vi "Trigger 2.vi"() -> ()   [LabVIEW 2012]
panel:
  in  "CO2 ppm":dbl(slide)
  in  "CO2 Trigger":T1={"Boost A Threshold"=0.0, "Boost A Hyst"=-250.0, "Boost B Threshold"=50.0, "Boost B Hyst"=-150.0}
  out "Alt Diff Down":bool
  out "Alt Dif Last":dbl
  out "Alt States":T2={"Main"=TRUE, "Boost A"=FALSE, "Boost B"=FALSE, "Recirc"=FALSE, "Scrubber"=FALSE, "O2 Valve"=FALSE, "Vent"=FALSE, "Alarm"=FALSE}
  in  "Alt Dif":dbl(slide) scale=-1000.0..1000.0
  in  "Stop Progam":bool
  out "Loops":i32
  in  "Alt Trigger":T3={"Boost A Threshold"=0.0, "Boost A Hyst"=-250.0, "Boost B Threshold"=50.0, "Boost B Hyst"=-150.0, "O2 Threshold"=250.0, "O2 Hyst"=400.0, "Vent Threshold"=50.0, "Vent Hyst"=200.0, "Recirc Threshold "=50.0, "Recirc  Hyst "=-150.0}
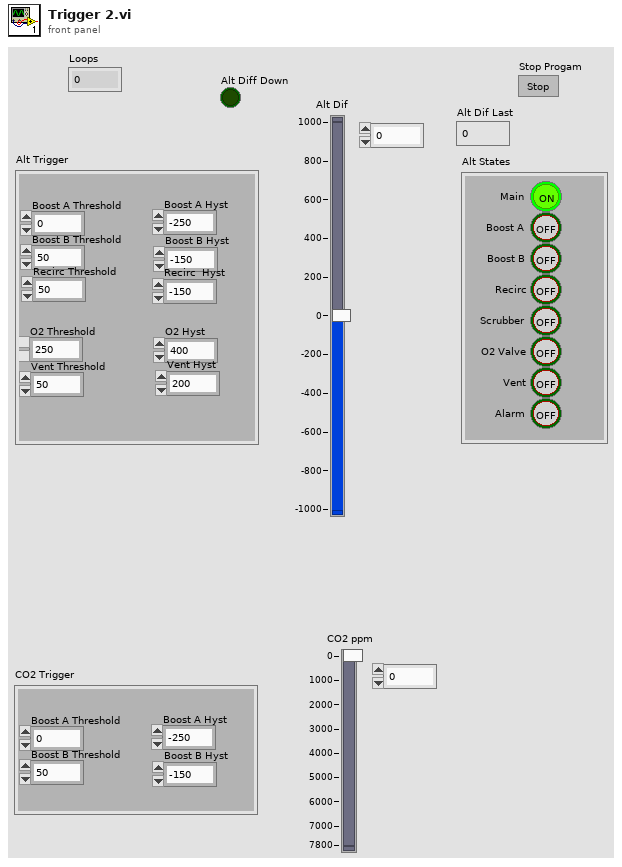
[diagram p1: front panel]
types:
  T1 = cluster{"Boost A Threshold":dbl, "Boost A Hyst":dbl, "Boost B Threshold":dbl, "Boost B Hyst":dbl}
  T2 = cluster{"Main":bool, "Boost A":bool, "Boost B":bool, "Recirc":bool, "Scrubber":bool, "O2 Valve":bool, "Vent":bool, "Alarm":bool}
  T3 = cluster{"Boost A Threshold":dbl, "Boost A Hyst":dbl, "Boost B Threshold":dbl, "Boost B Hyst":dbl, "O2 Threshold":dbl, "O2 Hyst":dbl, "Vent Threshold":dbl, "Vent Hyst":dbl, "Recirc Threshold ":dbl, "Recirc  Hyst ":dbl}
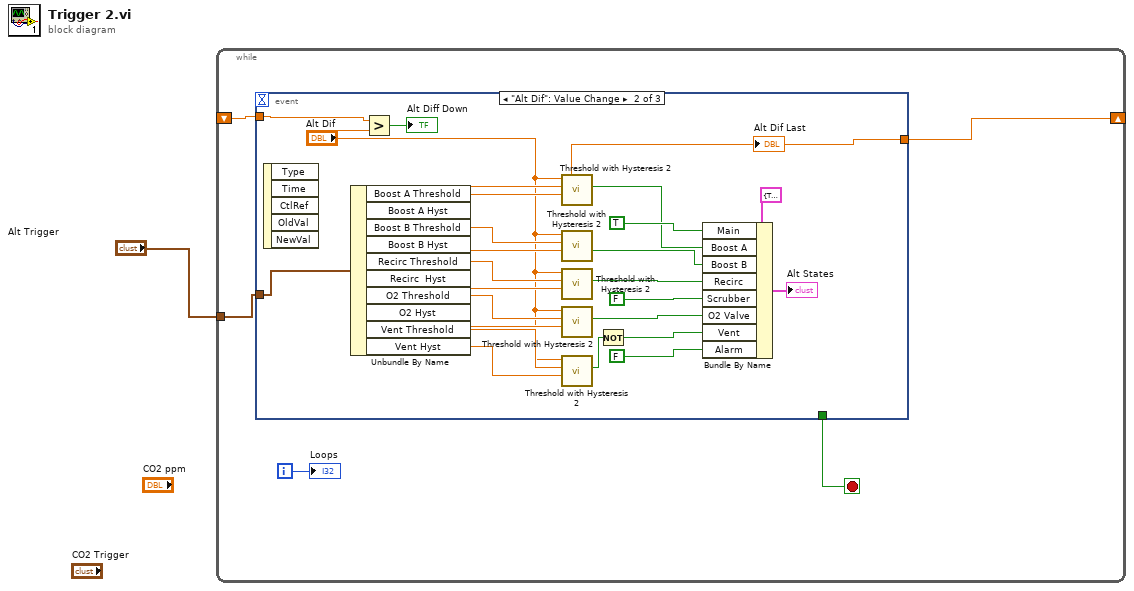
[diagram p0: block diagram]
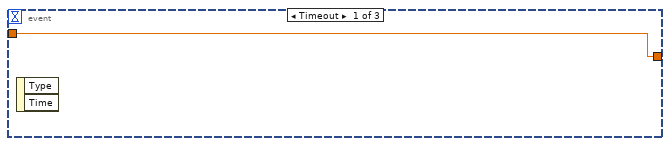
[diagram p2: hidden frame]
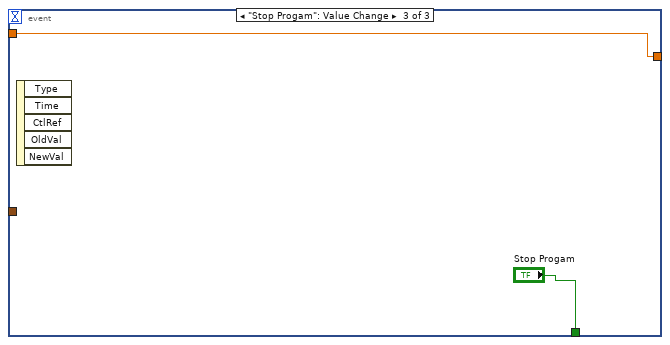
[diagram p3: hidden frame]
diagram:
  n1 = while {
    tunnel: "Alt Trigger" -> [w6]
    shift-right: [w3] -> _
    shift-left: _ -> [w4]
    i -> [w5]
    stop <- w2 stop-if-true
    n2 = event shown="[1] \"Alt Dif\": Value Change" {
      selector: _ -> [_ _ _]
      dyn-events: _ -> [_ _ _]
      timeout: _ -> [_ _ _]
      tunnel: w6 -> [_ w8 _]
      tunnel: w4 -> [w7 w9 w35]
      tunnel: [w7 w10 w35] -> w3
      tunnel: [_ _ "Stop Progam"] -> w2
      event Timeout {
        n3 = event-data() -> ()  [unwired: 1 in, 2 out]
      }
      event "Alt Dif": Value Change {
        n4 = event-data() -> ()  [unwired: 1 in, 5 out]
        n5 = Unbundle By Name(w8) -> ("Boost A Threshold"=w27:dbl, "Boost A Hyst"=w26:dbl, "Boost B Threshold"=w19:dbl, "Boost B Hyst"=w20:dbl, "Recirc Threshold"=w21:dbl, "Recirc  Hyst"=w22:dbl, "O2 Threshold"=w16:dbl, "O2 Hyst"=w15:dbl, "Vent Threshold"=w24:dbl, "Vent Hyst"=w23:dbl)
        n6 = Greater?(x=w9, y="Alt Dif") -> (0:→"Alt Diff Down":bool)
        n7 = call "Threshold with Hysteresis 2.vi"("Hystersis"=w26, "Threshold"=w27, "Input Dif"="Alt Dif") -> ("Power"=w14:bool, "Out Dif Last"=w10:dbl)  [unwired: 2 in, 2 out]
        "Alt Dif Last" <- w10
        n8 = call "Threshold with Hysteresis 2.vi"("Hystersis"=w20, "Threshold"=w19, "Input Dif"="Alt Dif") -> ("Threshold"=w25:bool)  [unwired: 2 in, 3 out]
        n9 = call "Threshold with Hysteresis 2.vi"("Hystersis"=w22, "Threshold"=w21, "Input Dif"="Alt Dif") -> ("Power"=w18:bool)  [unwired: 2 in, 3 out]
        n10 = call "Threshold with Hysteresis 2.vi"("Hystersis"=w15, "Threshold"=w16, "Input Dif"="Alt Dif") -> ("Power"=w17:bool)  [unwired: 2 in, 3 out]
        n11 = call "Threshold with Hysteresis 2.vi"("Hystersis"=w23, "Threshold"=w24, "Input Dif"="Alt Dif") -> ("Power"=w13:bool)  [unwired: 2 in, 3 out]
        n12 = Not(x=w13) -> (.not. x?=w28:bool)
        n13 = Bundle By Name(cluster=T2 {"Main"=TRUE, "Boost A"=FALSE, "Boost B"=FALSE, "Recirc"=FALSE, "Scrubber"=FALSE, "O2 Valve"=FALSE, "Vent"=FALSE, "Alarm"=FALSE} ("Alt States"), "Main"=TRUE, "Boost A"=w14, "Boost B"=w25, "Recirc"=w18, "Scrubber"=FALSE, "O2 Valve"=w17, "Vent"=w28, "Alarm"=FALSE) -> (→"Alt States":T2)
      }
      event "Stop Progam": Value Change {
        n14 = event-data() -> ()  [unwired: 1 in, 5 out]
      }
    }
    "Loops" <- w5
  }
